vi "roboRIO v1.0 Reserve IRQ.vi"(4 "Callback VI Ref":T1, 5 "Allow Overwrite? (F)":bool, 7 "Is Reserve?":bool, 8 "error in (no error)":errorcluster, 9 "IO IRQ Channels Enum":T3, 10 "IRQ Type":T2, 11 "IRQ Number":u8) -> (0 "error out":errorcluster, 2 "Succeed?":bool)   [LabVIEW 2021]
uses:
  <vilib>/myRIO/Common/Instrument Driver Framework/myRIO v1.0/IRQ/typedefs/IO IRQ Channels Enum.ctl
  <vilib>/myRIO/Common/Instrument Driver Framework/myRIO v1.0/IRQ/typedefs/IRQ Type.ctl
  <vilib>/myRIO/Common/Instrument Driver Framework/myRIO v1.0/IRQ/typedefs/Callback VI Ref.ctl
  <vilib>/myRIO/Common/Instrument Driver Framework/Utilities/typedefs/FPGA Ref Manager Action Enum.ctl
  <vilib>/myRIO/Common/Instrument Driver Framework/roboRIO v1.0/IRQ/typedefs/roboRIO Timer IRQ FPGA Reference.ctl
  <vilib>/myRIO/Common/Instrument Driver Framework/myRIO v1.0/IRQ/typedefs/Generic IRQ.ctl
  <vilib>/rvi/errors/niLvFpgaAdjustHostInterfaceError.vi
  <vilib>/rvi/interface/nirviReadWriteControl/nirviReadWriteControl.xnode
  NiFpgaLv.dll
  <vilib>/rvi/interface/Simulation/niFpgaSimulationCallBeginRW.vi
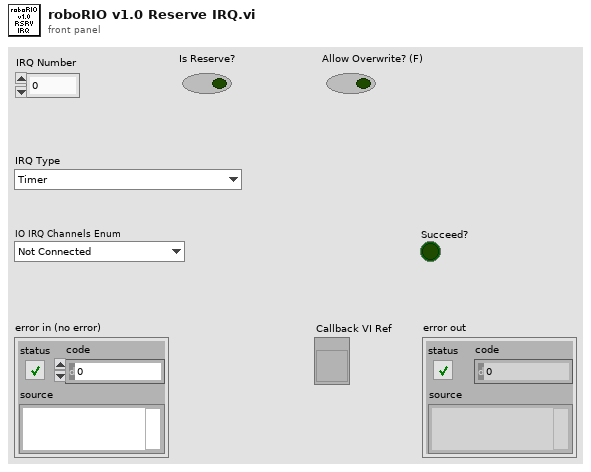
[diagram p1: front panel]
types:
  T1 = typedef "Callback VI Ref.ctl" = refnum<vi>
  T2 = typedef "IRQ Type.ctl" = enum16{"Timer", "Analog falling edge", "Analog rising edge", "Digital falling edge", "Digital rising edge", "Digital edge"}
  T3 = typedef "IO IRQ Channels Enum.ctl" = enum16{"Not Connected", "A/AI0 (Interrupt)", "A/AI1 (Interrupt)", "A/DIO0 (Interrupt)", "A/DIO1 (Interrupt)", "A/DIO2 (Interrupt)", "A/DIO3 (Interrupt)", "Button0 (Interrupt)", "B/AI0 (Interrupt)", "B/AI1 (Interrupt)", "B/DIO0 (Interrupt)", "B/DIO1 (Interrupt)", "B/DIO2 (Interrupt)", "B/DIO3 (Interrupt)"}
  T4 = typedef "FPGA Ref Manager Action Enum.ctl" = enum16{"Get", "Set", "Reset"}
  T5 = typedef "Generic IRQ.ctl" = cluster{"IRQ Type":T2, "IO IRQ Channels Enum":T3, "Callback VI Ref":T1, "Allow Overwrite?":bool, "Interrupt enabled?":bool}
  T6 = typedef "Generic IRQ Array.ctl" = T5[]
  T7 = typedef "Generic FPGA Reference.ctl" = refnum<k20>
  T8 = typedef "roboRIO Timer IRQ FPGA Reference.ctl" = refnum<k20>
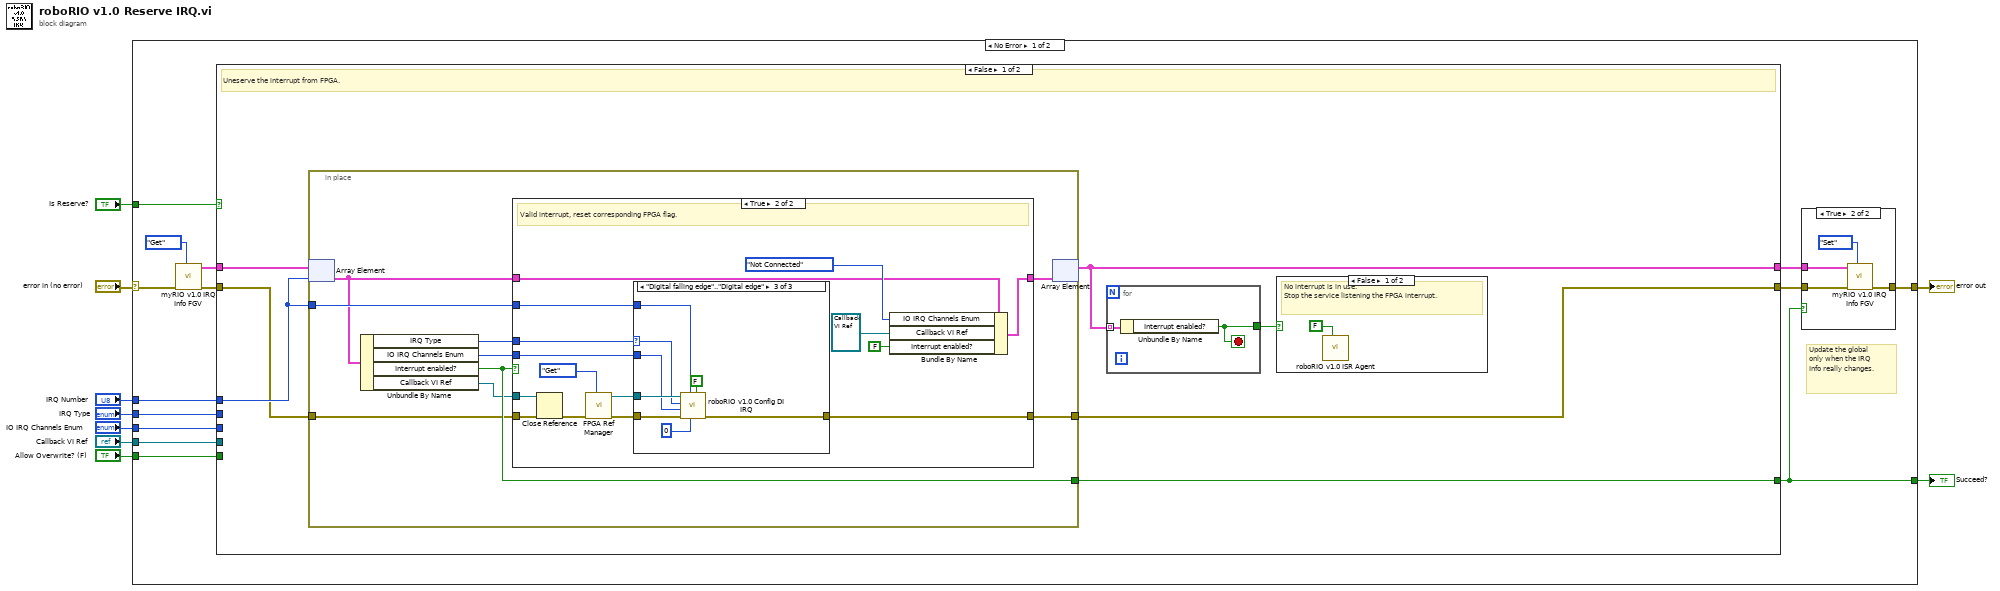
[diagram p0: block diagram]
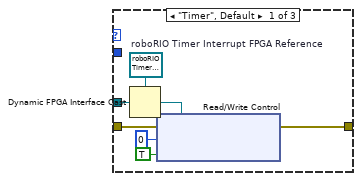
[diagram p4: hidden frame]
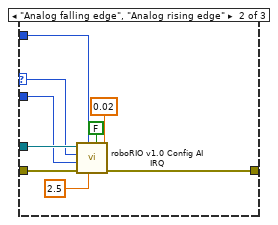
[diagram p5: hidden frame]
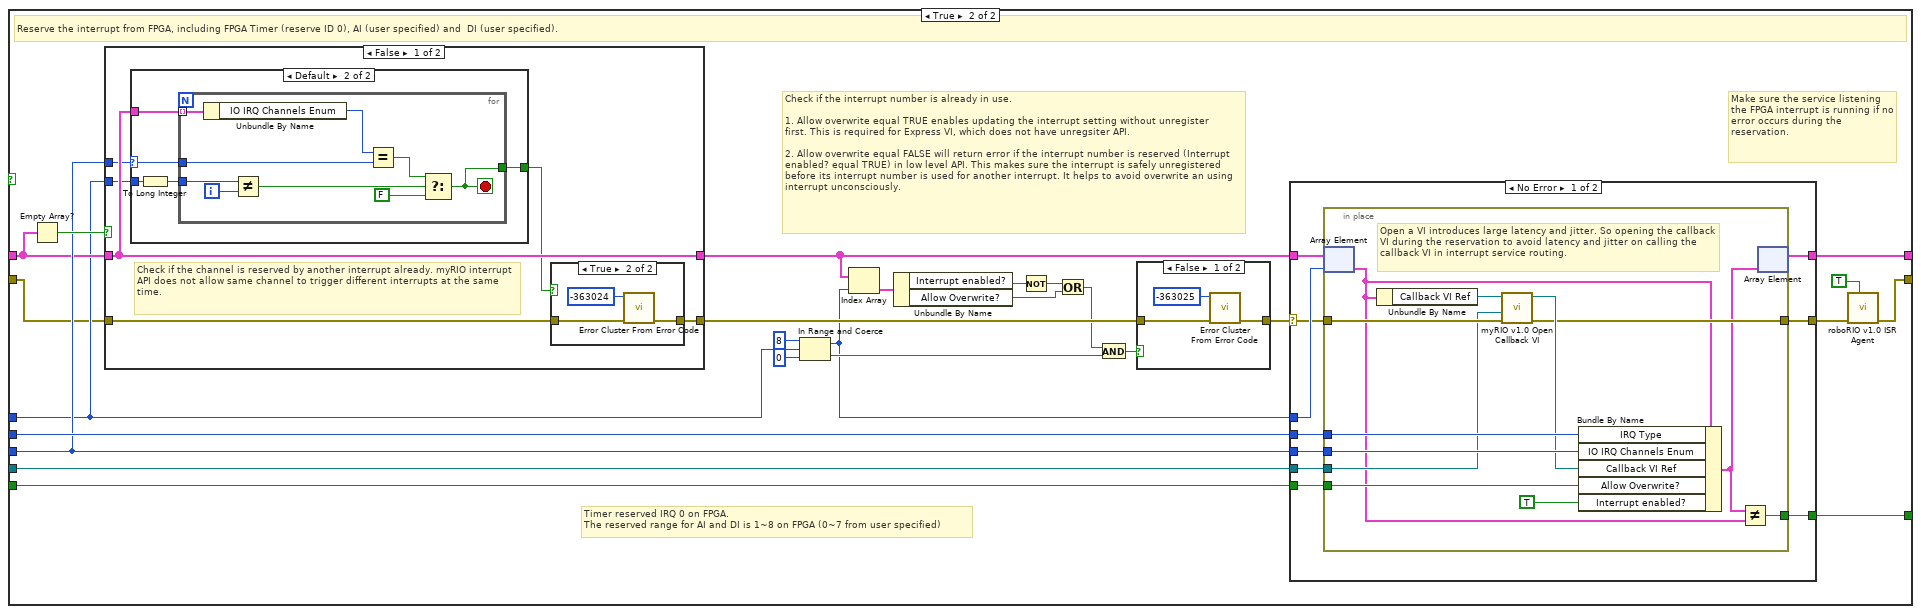
[diagram p6: hidden frame]
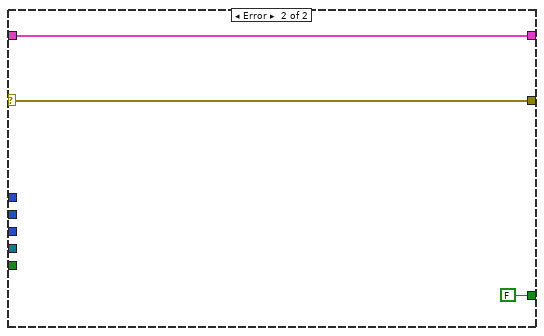
[diagram p8: hidden frame]
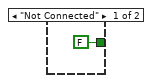
[diagram p10: hidden frame]
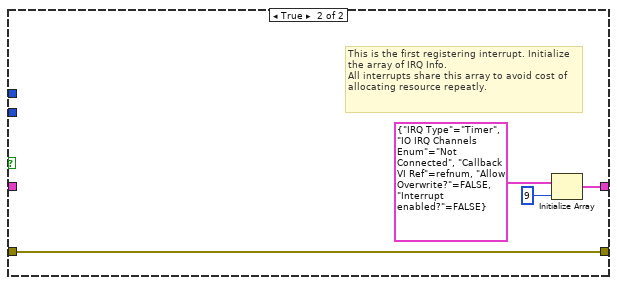
[diagram p11: hidden frame]
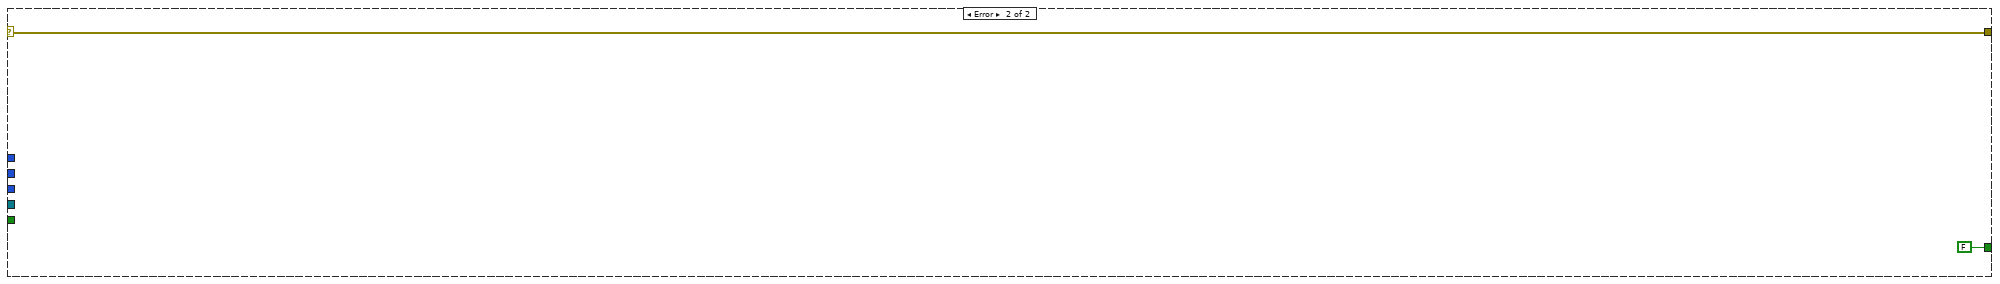
[diagram p13: hidden frame]
diagram:
  n1 = case shown="No Error" "error in (no error)" {
    selector: "error in (no error)" -> [w10 w173]
    tunnel: "IRQ Type" -> [w23 _]
    tunnel: "Callback VI Ref" -> [w22 _]
    tunnel: "Allow Overwrite? (F)" -> [w21 _]
    tunnel: [w20 w173] -> w6
    tunnel: "IO IRQ Channels Enum" -> [w19 _]
    tunnel: "IRQ Number" -> [w16 _]
    tunnel: [w13 FALSE ("Interrupt enabled?")] -> w3
    tunnel: "Is Reserve?" -> [w11 _]
    frame No Error {
      # "Update the global only when the IRQ Info really changes."
      n2 = call <vilib>:"myRIO v1.0 IRQ Info FGV.vi"("Action"=FPGA_Ref_Manager_Action_Enum."Get", "error in (no error)"=w10) -> ("error out"=w12:errorcluster, "Generic IRQ Info out"=w18:T6)  [unwired: 8 in]
      n3 = case shown="False" w11 {
        tunnel: w23 -> [_ w109]
        tunnel: w22 -> [_ w108]
        tunnel: w21 -> [_ w106]
        tunnel: w19 -> [_ w105]
        tunnel: w18 -> [w28 w104]
        tunnel: w16 -> [w29 w90]
        tunnel: [w26 w89] -> w15
        tunnel: [w24 w84] -> w14
        tunnel: [w25 w88] -> w13
        tunnel: w12 -> [w27 w87]
        frame False {
          # "Uneserve the interrupt from FPGA."
          n4 = in-place {
            in-place-border: [w41] -> w25
            in-place-border: w29 -> [w39]
            in-place-border: w27 -> [w37]
            in-place-border: [w36] -> w24
            n5 = in-place-array #1(w28, w29) -> (w34:T5)
            n6 = Unbundle By Name(w34) -> ("IRQ Type"=w40:T2, "IO IRQ Channels Enum"=w38:T3, "Interrupt enabled?"=w41:bool, "Callback VI Ref"=w35:T1)
            n7 = case shown="True" w41 {
              tunnel: [w44 w59] -> w42
              tunnel: w34 -> [w44 w55]
              tunnel: w40 -> [_ w54]
              tunnel: w39 -> [_ w51]
              tunnel: w38 -> [_ w50]
              tunnel: w37 -> [w43 w47]
              tunnel: [w43 w48] -> w36
              tunnel: w35 -> [_ w45]
              frame False {
                # "Invalid interrupt, do nothing."
              }
              frame True {
                # "Valid interrupt, reset corresponding FPGA flag."
                n8 = Close Reference(reference=w45, error in (no error)=w47) -> (error out=w46:errorcluster)
                n9 = call <vilib>:"FPGA Ref Manager.vi"("Action"=FPGA_Ref_Manager_Action_Enum."Get", "error in (no error)"=w46) -> ("error out"=w49:errorcluster, "Generic FPGA Reference out"=w52:T7)  [unwired: 7 in]
                n10 = case shown="\"Digital falling edge\"..\"Digital edge\"" w54 {
                  selector: w54 -> [_ w72 w80]
                  tunnel: w52 -> [w63 w75 w81]
                  tunnel: w51 -> [_ w74 w82]
                  tunnel: w50 -> [_ w71 w79]
                  tunnel: w49 -> [w62 w70 w78]
                  tunnel: [w61 w68 w77] -> w48
                  frame "Timer", Default {
                    w60 = T8 refnum  # roboRIO Timer Interrupt FPGA Reference
                    n11 = Dynamic FPGA Interface Cast(Session In=w60, Type=w63) -> (Session Out=w66:T8)
                    n12 = xnode "Read/Write Control"("FPGA VI Reference In"=w66, "error in"=w62, "IRQ.TIMER.WRITE"=u32 0 ("Timeout"), "IRQ.TIMER.SETTIME"=TRUE ("TIMER.SetTime")) -> ("error out"=w61:errorcluster)  [unwired: 1 out]
                  }
                  frame "Analog falling edge", "Analog rising edge" {
                    n13 = call <vilib>:"roboRIO v1.0 Config AI IRQ.vi"("Hysteresis"=0.02, "Enable IRQ?"=FALSE, "Threshold"=2.5, "IRQ Number"=w74, "error in (no error)"=w70, "IO IRQ Channels Enum"=w71, "IRQ Type"=w72, "myRIO FPGA Ref In"=w75) -> ("error out"=w68:errorcluster)  [unwired: 3 in]
                  }
                  frame "Digital falling edge".."Digital edge" {
                    n14 = call <vilib>:"roboRIO v1.0 Config DI IRQ.vi"("Enable IRQ?"=FALSE, "Edge Count"=u32 0, "IRQ Number"=w82, "error in (no error)"=w78, "IO IRQ Channels Enum"=w79, "IRQ Type"=w80, "myRIO FPGA Ref In"=w81) -> ("error out"=w77:errorcluster)  [unwired: 4 in]
                  }
                }
                n15 = Bundle By Name(cluster=w55, "IO IRQ Channels Enum"=IO_IRQ_Channels_Enum."Not Connected", "Callback VI Ref"=T1 refnum, "Interrupt enabled?"=FALSE) -> (w59:T5)
              }
            }
            n16 = in-place-array #1(w42) -> (w26:T6)  [unwired: 1 out]
          }
          n17 = for {
            tunnel: w26 -> [w33] mode=indexing
            tunnel: [w32] -> w30
            stop <- w32 stop-if-true
            n18 = Unbundle By Name(w33) -> ("Interrupt enabled?"=w32:bool)
          }
          n19 = case shown="False" w30 {
            frame False {
              # "No interrupt is in use.\nStop the service listening the FPGA interrupt."
              n20 = call <vilib>:"roboRIO v1.0 ISR Agent.vi"("Run?"=FALSE) -> ()  [unwired: 10 in, 1 out]
            }
            frame True {
              # "There is interrupt still in use. Do nothing."
            }
          }
        }
        frame True {
          # "Make sure the service listening the FPGA interrupt is running if no error occurs during the reservation."
          # "Check if the interrupt number is already in use.\n\n1. Allow overwrite equal TRUE enables updating the interrupt setting without unregister\nfirst. This is required for Express VI, which does not have unregsiter API.\n\n2. Allow overwrite equal FALSE will return error if the interrupt number is reserved (Interrupt enabled? equal TRUE) in low level API. This makes sure the interrupt is safely unregistered before its interrupt number is used for another interrupt. It helps to avoid overwrite an using interrupt unconsciously."
          # "Timer reserved IRQ 0 on FPGA. \nThe reserved range for AI and DI is 1~8 on FPGA (0~7 from user specified)"
          # "Reserve the interrupt from FPGA, including FPGA Timer (reserve ID 0), AI (user specified) and  DI (user specified)."
          n21 = Empty Array?(array=w104) -> (empty?=w107:bool)
          n22 = case shown="False" w107 {
            tunnel: [w144 w165] -> w96
            tunnel: w104 -> [w144 _]
            tunnel: [w141 w164] -> w97
            tunnel: w105 -> [w143 _]
            tunnel: w90 -> [w140 _]
            tunnel: w87 -> [w139 w164]
            frame False {
              # "Check if the channel is reserved by another interrupt already. myRIO interrupt API does not allow same channel to trigger different interrupts at the same time."
              n23 = case shown="Default" w143 {
                selector: w143 -> [_ w154]
                tunnel: w144 -> [_ w150]
                tunnel: [FALSE w153] -> w142
                tunnel: w140 -> [_ w152]
                frame "Not Connected" {
                }
                frame Default {
                  n24 = To Long Integer(number=w152) -> (32bit integer=w151:i32)
                  n25 = for {
                    tunnel: w154 -> [w162]
                    tunnel: [w156] -> w153
                    tunnel: w151 -> [w160]
                    tunnel: w150 -> [w155] mode=indexing
                    i -> [w161]
                    stop <- w156 stop-if-true
                    n26 = Unbundle By Name(w155) -> ("IO IRQ Channels Enum"=w163:T3)
                    n27 = Not Equal?(x=w160, y=w161) -> (x != y?=w159:bool)
                    n28 = Equal?(x=w163, y=w162) -> (x = y?=w157:bool)
                    n29 = Select(t=w157, s=w159, f=FALSE) -> (s? t:f=w156:bool)
                  }
                }
              }
              n30 = case shown="True" w142 {
                tunnel: [w145 w147] -> w141
                tunnel: w139 -> [w145 w146]
                frame False {
                }
                frame True {
                  n31 = call <vilib>:"Error Cluster From Error Code.vi"("error in (no error)"=w146, "error code (0)"=-363024) -> ("error out"=w147:errorcluster)  [unwired: 7 in]
                }
              }
            }
            frame True {
              # "This is the first registering interrupt. Initialize the array of IRQ Info. \nAll interrupts share this array to avoid cost of allocating resource repeatly."
              n32 = Initialize Array(T5 {"IRQ Type"=enum."Timer", "IO IRQ Channels Enum"=enum."Not Connected", "Callback VI Ref"=refnum, "Allow Overwrite?"=FALSE, "Interrupt enabled?"=FALSE} ("Interrupt Info"), 9 ("dimension size")) -> (w165:T5[])
            }
          }
          n33 = In Range and Coerce(upper limit=u8 8, x=w90, lower limit=u8 0) -> (coerced(x)=w91:u8, In Range?=w93:bool)
          n34 = Index Array(array=w96, index=w91) -> (element=w98:T5)
          n35 = Unbundle By Name(w98) -> ("Interrupt enabled?"=w99:bool, "Allow Overwrite?"=w101:bool)
          n36 = Not(x=w99) -> (.not. x?=w100:bool)
          n37 = Or(x=w100, y=w101) -> (x .or. y?=w94:bool)
          n38 = And(x=w94, y=w93) -> (x .and. y?=w92:bool)
          n39 = case shown="False" w92 {
            tunnel: [w111 w113] -> w95
            tunnel: w97 -> [w110 w113]
            frame False {
              n40 = call <vilib>:"Error Cluster From Error Code.vi"("error in (no error)"=w110, "error code (0)"=-363025) -> ("error out"=w111:errorcluster)  [unwired: 7 in]
            }
            frame True {
            }
          }
          n41 = case shown="No Error" w95 {
            selector: w95 -> [w116 w137]
            tunnel: w105 -> [w123 _]
            tunnel: w109 -> [w122 _]
            tunnel: w108 -> [w121 _]
            tunnel: [w120 w138] -> w89
            tunnel: w96 -> [w119 w138]
            tunnel: w106 -> [w118 _]
            tunnel: w91 -> [w117 _]
            tunnel: [w115 w137] -> w85
            tunnel: [w114 FALSE] -> w88
            frame No Error {
              n42 = in-place {
                in-place-border: w121 -> [w127]
                in-place-border: w122 -> [w135]
                in-place-border: w123 -> [w134]
                in-place-border: w118 -> [w133]
                in-place-border: w116 -> [w130]
                in-place-border: [w129] -> w115
                in-place-border: [w124] -> w114
                # "Open a VI introduces large latency and jitter. So opening the callback VI during the reservation to avoid latency and jitter on calling the callback VI in interrupt service routing."
                n43 = in-place-array #2(w119, w117) -> (w125:T5)
                n44 = Unbundle By Name(w125) -> ("Callback VI Ref"=w128:T1)
                n45 = call <vilib>:"myRIO v1.0 Open Callback VI.vi"("error in (no error)"=w130, "Static Ref in"=w127, "Opened VI Ref in"=w128) -> ("error out"=w129:errorcluster, "Opened VI Ref out"=w131:T1)  [unwired: 7 in]
                n46 = Bundle By Name(cluster=w125, "IRQ Type"=w135, "IO IRQ Channels Enum"=w134, "Callback VI Ref"=w131, "Allow Overwrite?"=w133, "Interrupt enabled?"=TRUE) -> (w126:T5)
                n47 = Not Equal?(x=w126, y=w125) -> (x != y?=w124:bool)
                n48 = in-place-array #2(w126) -> (w120:T6)  [unwired: 1 out]
              }
            }
            frame Error {
            }
          }
          n49 = call <vilib>:"roboRIO v1.0 ISR Agent.vi"("Run?"=TRUE, "error in (no error)"=w85) -> ("error out"=w84:errorcluster)  [unwired: 9 in]
        }
      }
      n50 = case shown="True" w13 {
        tunnel: [w168 w172] -> w20
        tunnel: w15 -> [_ w170]
        tunnel: w14 -> [w168 w169]
        frame False {
        }
        frame True {
          n51 = call <vilib>:"myRIO v1.0 IRQ Info FGV.vi"("Action"=FPGA_Ref_Manager_Action_Enum."Set", "error in (no error)"=w169, "Generic IRQ Info in"=w170) -> ("error out"=w172:errorcluster)  [unwired: 7 in, 1 out]
        }
      }
    }
    frame Error {
    }
  }
  "error out" <- w6
  "Succeed?" <- w3
